vi "Actor Core.vi"(8 "error in":errorcluster, 11 "CRIO MSS Test Actor in":refnum<class "CRIO MSS Test Actor.lvclass">) -> (0 "error out":errorcluster, 3 "Actor out":refnum<class "Actor.lvclass">)   [LabVIEW 2023, in "CRIO MSS Test Actor.lvlib" / "CRIO MSS Test Actor.lvclass"]
doc: "(<B>Filename</B>: Actor Framework.lvlib:Actor.lvclass:Actor Core.vi)\n\nReceives messages to the actor, reacts to them, and initiates any error handling that may shut the actor down.\n\nDescendant classes may override this VI to append parallel tasks for the actor to complete while it handles messages. Overrides use the Call Parent Class Method node."
uses:
  CRIO MSS Test Actor.lvclass
  CRIO MSS Test Actor.lvclass/CRIO MSS Test Actor.ctl
  <vilib>/ActorFramework/Actor/Actor.lvclass
  <vilib>/ni/Actors/Network Endpoint Actors/Notifying Nested Endpoint/Notifying Nested Endpoint.lvclass
  <vilib>/ni/Actors/Network Endpoint Actors/Network Endpoint/Network Endpoint/Network Endpoint.lvclass
  C:/Program Files/National Instruments/LabVIEW 2023/vi.lib/ni/Actors/Network Endpoint Actors/Nested Endpoint/Nested Endpoint/Nested Endpoint.lvclass
  C:/Program Files/National Instruments/LabVIEW 2023/vi.lib/ni/Actors/Network Endpoint Actors/Network Endpoint/Network Endpoint/Network Endpoint.lvclass
  C:/Program Files/National Instruments/LabVIEW 2023/vi.lib/ActorFramework/Actor/Actor.lvclass
  C:/Program Files/National Instruments/LabVIEW 2023/vi.lib/ni/Actors/Network Endpoint Actors/Notifying Nested Endpoint/Notifying Nested Endpoint.lvclass
  D:/git/HAL/HAL GOOP4/Host Measure and Stimulus Subsystems/Tests/CRIO MSS Test Actor/CRIO MSS Test Actor/CRIO MSS Test Actor.lvclass
  D:/git/HAL/HAL GOOP4/Host Measure and Stimulus Subsystems/Tests/CRIO MSS Test Actor/ICRIO MSS Test Actor/ICRIO MSS Test Actor.lvclass
  C:/Program Files/National Instruments/LabVIEW 2023/vi.lib/ni/Actors/Network Endpoint Actors/Nested Endpoint Caller/Nested Endpoint Caller/Nested Endpoint Caller.lvclass
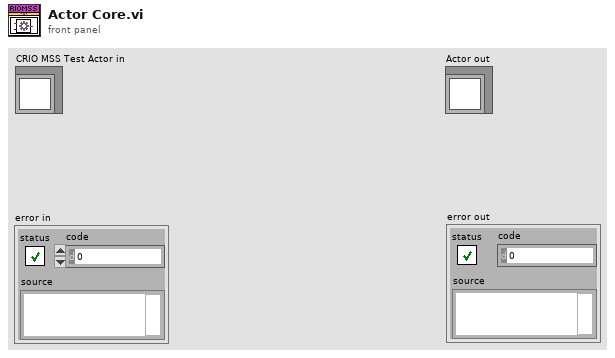
[diagram p1: front panel]
types:
  T1 = map{string, refnum<class "Message Enqueuer.lvclass">}
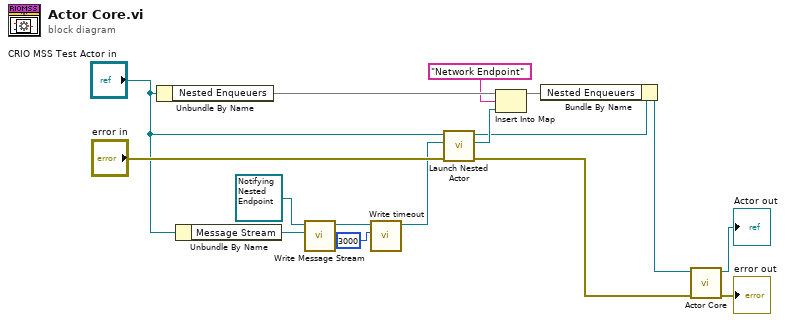
[diagram p0: block diagram]
diagram:
  n1 = Unbundle By Name("CRIO MSS Test Actor in") -> ("Nested Enqueuers"=w6:T1)
  n2 = Unbundle By Name("CRIO MSS Test Actor in") -> ("Message Stream"=w11:refnum<class "Message Stream.lvclass">)
  n3 = call <vilib>:"Write Message Stream.vi"("Message Stream"=w11, "Network Endpoint in"=refnum<class "Notifying Nested Endpoint.lvclass"> refnum ("Notifying Nested Endpoint.lvclass")) -> ("Network Endpoint out"=w12:refnum<class "Notifying Nested Endpoint.lvclass">)  [unwired: 9 in]
  n4 = call <vilib>:"Write timeout.vi"("timeout"=3000, "Network Endpoint in"=w12) -> ("Network Endpoint out"=w8:refnum<class "Notifying Nested Endpoint.lvclass">)  [unwired: 9 in]
  n5 = call <vilib>:"Launch Nested Actor.vi"("error in (no error)"="error in", "Nested Actor"=w8, "Caller Actor in"="CRIO MSS Test Actor in") -> ("error out"=w9:errorcluster, "Nested Actor's Enqueuer"=w4:refnum<class "Message Enqueuer.lvclass">, "Caller Actor out"=w3:refnum<class "CRIO MSS Test Actor.lvclass">)  [unwired: 6 in]
  n6 = Insert Into Map(map in=w6, key="Network Endpoint", value=w4) -> (map out=w1:T1)  [unwired: 2 out]
  n7 = Bundle By Name(cluster=w3, "Nested Enqueuers"=w1) -> (w2:refnum<class "CRIO MSS Test Actor.lvclass">)
  n8 = call-parent "Actor Core.vi"("error in"=w9, "Actor in"=w2) -> ("error out"=→"error out":errorcluster, "Actor out"=→"Actor out":refnum<class "Actor.lvclass">)  [unwired: 8 in]
